vi "软件系统框架.vi"   [LabVIEW 2017]
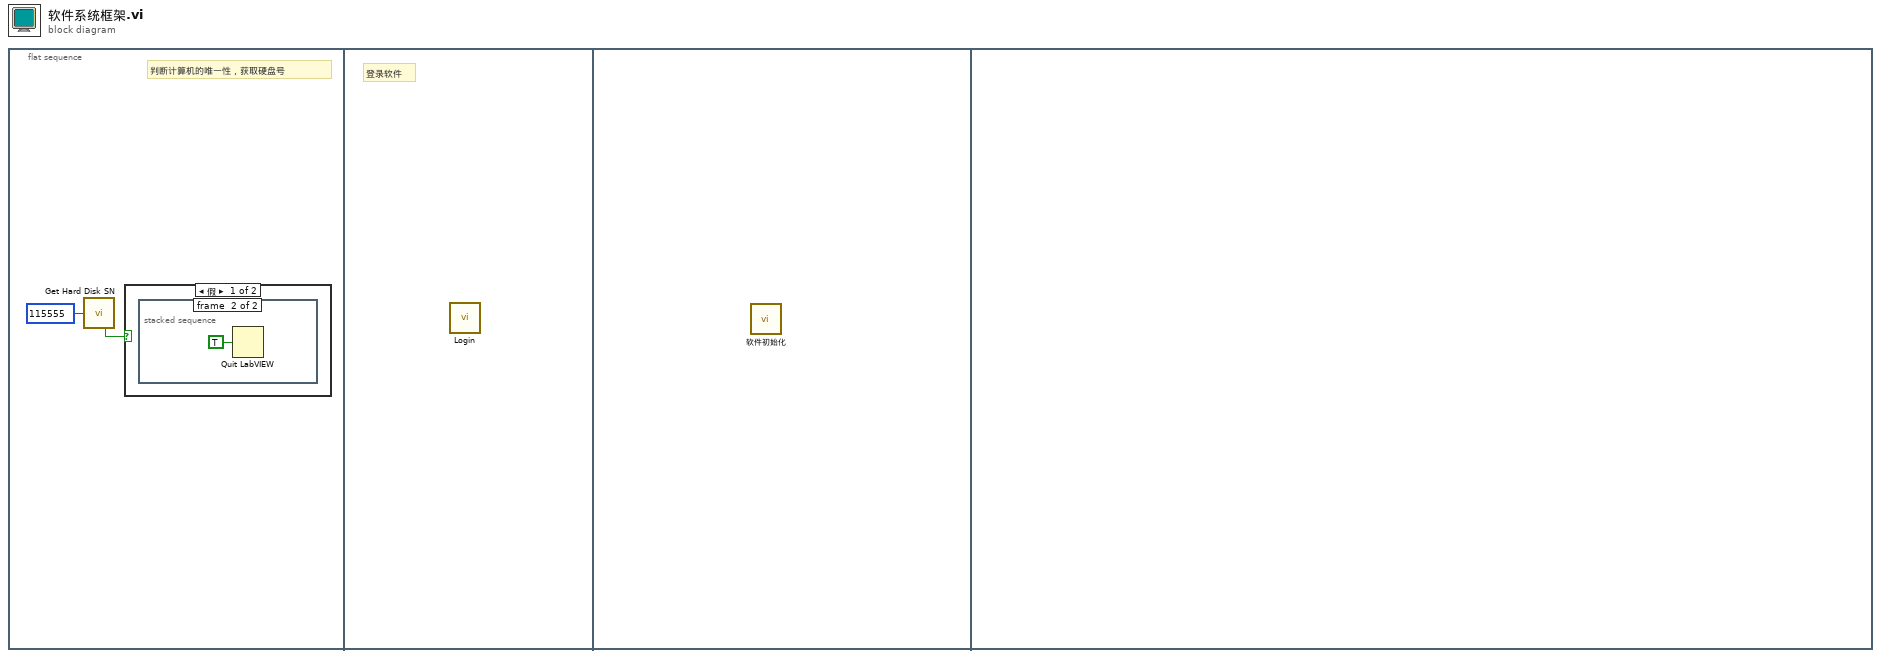
[diagram p0: block diagram]
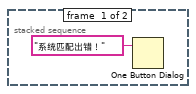
[diagram p2: hidden frame]
diagram:
  n1 = flat-sequence {
    frame #0 {
      # "判断计算机的唯一性，获取硬盘号"
      n2 = call "Get Hard Disk SN.vi"("当前D盘ID"=u32 115555) -> ("系统匹配？"=w2:bool)  [unwired: 9 in, 5 out]
      n3 = case shown="假" w2 {
        frame False {
          n4 = stacked-sequence {
            frame #0 {
              n5 = One Button Dialog(message="系统匹配出错！" ("消息")) -> ()  [unwired: 1 in, 1 out]
            }
            frame #1 {
              n6 = Quit LabVIEW(quit? (T)=TRUE ("退出？(T)")) -> ()
            }
          }
        }
        frame True {
        }
      }
    }
    frame #1 {
      # "登录软件"
      n7 = call "Login.vi"() -> ()  [unwired: 1 in]
    }
    frame #2 {
      n8 = call "软件初始化.vi"() -> ()  [unwired: 12 in]
    }
    frame #3 {
    }
  }
